vi "CheckNodeName.vi"(3 "node":string) -> (0 "New Node?":bool, 1 "Node":cluster{"name":string, "Port":u16})   [LabVIEW 2012]
doc: "Checks the node name and opens a new node if the name does not exist"
uses:
  _ROSDefinition.vi
  _ROSDirection.ctl
  _ROSControl.ctl
panel:
  out "compare":string
  out "checked":string[](array[string])
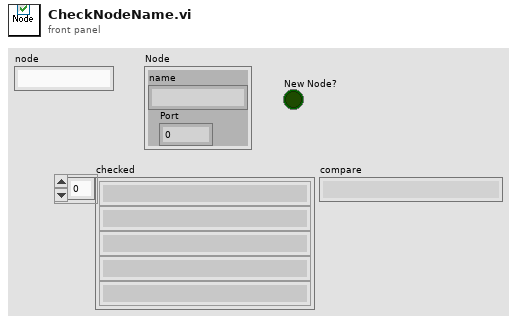
[diagram p1: front panel]
types:
  T1 = typedef "_ROSControl.ctl" = cluster{"topic port":u16, "Node":string, "topic":string, "type":string, "node port":u16, "error ":errorcluster, "Direction":T2, "Update (ms)":u16, "FIFO size":u16}
  T2 = typedef "_ROSDirection.ctl" = enum16{"Node", "Publisher", "Subscriber", "ServiceClient", "ServiceProvider"}
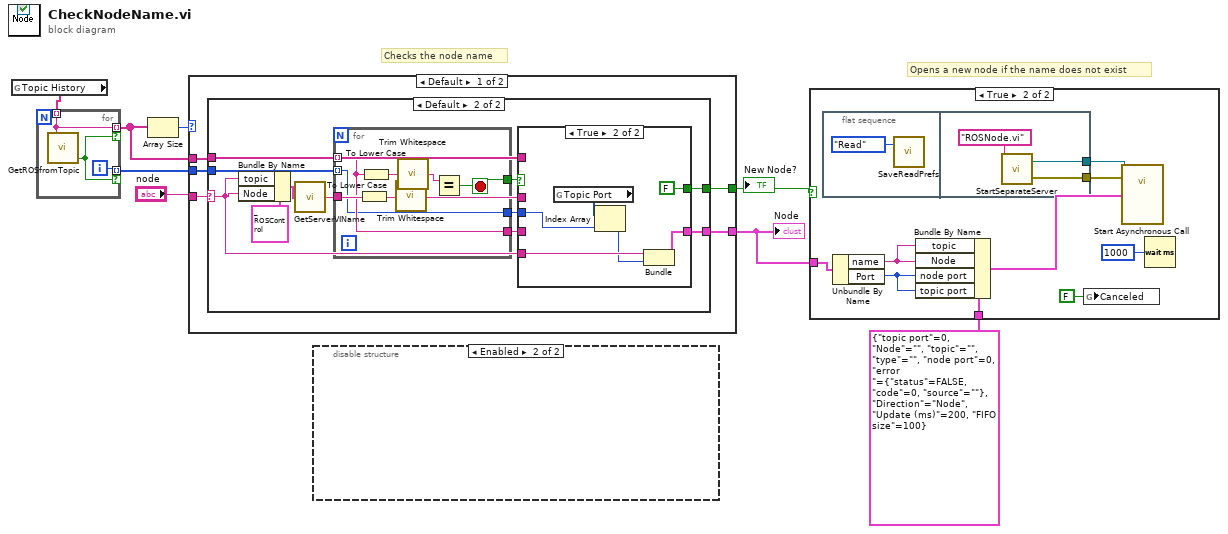
[diagram p0: block diagram]
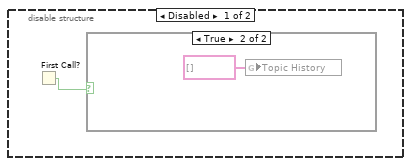
[diagram p2: hidden frame]
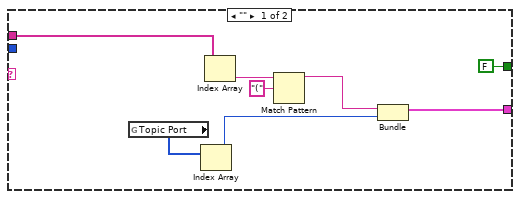
[diagram p4: hidden frame]
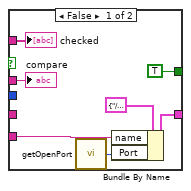
[diagram p5: hidden frame]
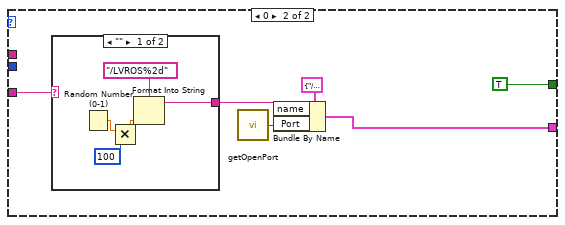
[diagram p6: hidden frame]
diagram:
  # "Opens a new node if the name does not exist"
  # "Checks the node name"
  n1 = global read "_ROSDefinition.vi" "Topic History"() -> (w3:string[])
  n2 = for {
    tunnel: w3 -> [w11] mode=indexing
    tunnel: [w11] -> w2 mode=indexing if=w9
    tunnel: [w10] -> w1 mode=indexing if=w9
    i -> [w10]
    n3 = call "GetROSfromTopic.vi"("Topic"=w11) -> ("Node?"=w9:bool)  [unwired: 2 in, 1 out]
  }
  n4 = Array Size(array=w2) -> (size(s)=w5:i32)
  n5 = case shown="Default" w5 {
    tunnel: "node" -> [w16 w62]
    tunnel: [w14 TRUE] -> w8
    tunnel: [w13 w57] -> w7
    tunnel: w2 -> [w15 _]
    tunnel: w1 -> [w12 _]
    frame Default {
      n6 = case shown="Default" w16 {
        selector: w16 -> [_ w25]
        tunnel: [w21 w35] -> w13
        tunnel: w15 -> [w17 w34]
        tunnel: [FALSE w31] -> w14
        tunnel: w12 -> [_ w26]
        frame "" {
          n7 = global read "_ROSDefinition.vi" "Topic Port"() -> (w23:u16[])
          n8 = Index Array(array=w23) -> (element=w22:u16)  [unwired: 1 in]
          n9 = Index Array(array=w17) -> (element=w19:string)  [unwired: 1 in]
          n10 = Match Pattern(string=w19, regular expression="(") -> (before substring=w18:string)  [unwired: 1 in, 3 out]
          n11 = Bundle("ROS Master"=w18, "Ports"=w22) -> (w21:cluster{"ROS Master":string, "Ports":u16})  [unwired: 1 in]
        }
        frame Default {
          n12 = Bundle By Name(cluster=T1 {"topic port"=0, "Node"="", "topic"="", "type"="", "node port"=0, "error "={"status"=FALSE, "code"=0, "source"=""}, "Direction"=enum."Node", "Update (ms)"=200, "FIFO size"=100} ("ROS"), "topic"=w25, "Node"=w25) -> (w28:T1)
          n13 = call "GetServerVIName.vi"("ROS"=w28) -> ("vi name"=w27:string)
          n14 = for {
            tunnel: w27 -> [w52]
            tunnel: [w54] -> w32
            tunnel: [w50] -> w33
            tunnel: w34 -> [w50] mode=indexing
            tunnel: [w49] -> w30
            tunnel: w26 -> [w49] mode=indexing
            stop <- w54 stop-if-true
            n15 = To Lower Case(string=w52) -> (all lower case string=w53:string)
            n16 = To Lower Case(string=w50) -> (all lower case string=w56:string)
            n17 = call <vilib>:"Trim Whitespace.vi"("string"=w53) -> ("trimmed string"=w51:string)  [unwired: 1 in]
            n18 = call <vilib>:"Trim Whitespace.vi"("string"=w56) -> ("trimmed string"=w55:string)  [unwired: 1 in]
            n19 = Equal?(x=w55, y=w51) -> (x = y?=w54:bool)
          }
          n20 = case shown="True" w32 {
            tunnel: [w41 w43] -> w35
            tunnel: w33 -> [_ _]
            tunnel: w34 -> [w37 _]
            tunnel: w25 -> [w42 w47]
            tunnel: [TRUE FALSE] -> w31
            tunnel: w30 -> [_ w46]
            tunnel: w27 -> [w36 _]
            frame False {
              n21 = call "getOpenPort.vi"() -> ("port"=w40:u16)
              n22 = Bundle By Name(cluster=cluster{"name":string, "Port":u16} {"name"="/LVROS", "Port"=0} ("Node"), "name"=w42, "Port"=w40) -> (w41:cluster{"name":string, "Port":u16})
              "checked" <- w37
              "compare" <- w36
            }
            frame True {
              n23 = global read "_ROSDefinition.vi" "Topic Port"() -> (w45:u16[])
              n24 = Index Array(array=w45, index=w46) -> (element=w44:u16)
              n25 = Bundle(w47, "Ports"=w44) -> (w43:cluster{string, "Ports":u16})  [unwired: 1 in]
            }
          }
        }
      }
    }
    frame 0 {
      n26 = case shown="\"\"" w62 {
        selector: w62 -> [_ w68]
        tunnel: [w63 w68] -> w59
        frame "" {
          n27 = Random Number (0-1)() -> (number: 0 to 1=w66:dbl)
          n28 = Multiply(x=w66, y=100) -> (x*y=w65:dbl)
          n29 = Format Into String(format string="/LVROS%2d" ("name"), w65) -> (resulting string=w63:string)  [unwired: 2 in, 1 out]
        }
        frame Default {
        }
      }
      n30 = call "getOpenPort.vi"() -> ("port"=w60:u16)
      n31 = Bundle By Name(cluster=cluster{"name":string, "Port":u16} {"name"="/LVROS", "Port"=0} ("Node"), "name"=w59, "Port"=w60) -> (w57:cluster{"name":string, "Port":u16})
    }
  }
  "Node" <- w7
  "New Node?" <- w8
  n32 = disable-structure shown="Enabled" {
    frame Disabled {
      n33 = First Call?() -> (First Call?: T/F=w69:bool)
      n34 = case shown="True" w69 {
        frame False {
        }
        frame True {
          n35 = global write "_ROSDefinition.vi" "Topic History"(string[] [] ("Topic History")) -> ()
        }
      }
    }
    frame Enabled {
    }
  }
  n36 = case shown="True" w8 {
    tunnel: w7 -> [_ w79]
    tunnel: T1 {"topic port"=0, "Node"="", "topic"="", "type"="", "node port"=0, "error "={"status"=FALSE, "code"=0, "source"=""}, "Direction"=enum."Node", "Update (ms)"=200, "FIFO size"=100} ("ROS") -> [_ w78]
    frame False {
    }
    frame True {
      n37 = flat-sequence {
        tunnel: [w82] -> w75
        tunnel: [w81] -> w74
        frame #0 {
          n38 = call "SaveReadPrefs.vi"("Task"=enum16{"Read", "Save"}."Read") -> ()  [unwired: 2 in, 1 out]
        }
        frame #1 {
          n39 = call "StartSeparateServer.vi"("Server"="ROSNode.vi") -> ("error out"=w82:errorcluster, "Ref out"=w81:refnum<vi>)  [unwired: 1 in]
        }
      }
      n40 = Unbundle By Name(w79) -> ("name"=w77:string, "Port"=w76:u16)
      n41 = Bundle By Name(cluster=w78, "topic"=w77, "Node"=w77, "node port"=w76, "topic port"=w76) -> (w73:T1)
      n42 = global write "_ROSDefinition.vi" "Canceled"(FALSE ("Canceled")) -> ()
      n43 = call-by-ref "Start Asynchronous Call"(reference=w74, error in=w75, "ROS"=w73) -> ()  [unwired: 3 in, 2 out]
      n44 = Wait (ms)(milliseconds to wait=u32 1000) -> ()  [unwired: 1 out]
    }
  }
